vi "alignTop.vi"(8 "error in (no error)":errorcluster, 11 "refs":refnum<vi>[](array[refnum])) -> (0 "error out":errorcluster, 3 "refs(dup)":refnum<vi>[](array[refnum]))   [LabVIEW 2023, in "TLC_Geometry.lvlib"]
doc: "Aligns all controls to the topmost position among the input controls.\nThe topmost coordinate is computed and applied to all controls."
uses:
  TLC_Geometry.lvlib
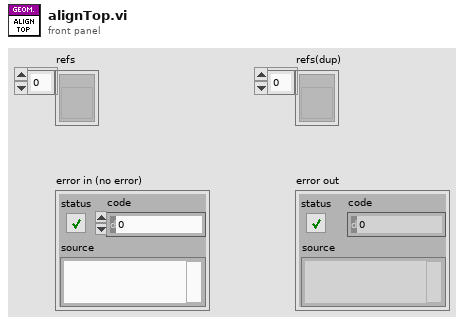
[diagram p1: front panel]
types:
  T1 = cluster{"left":i32, "top":i32, "right":i32, "bottom":i32}
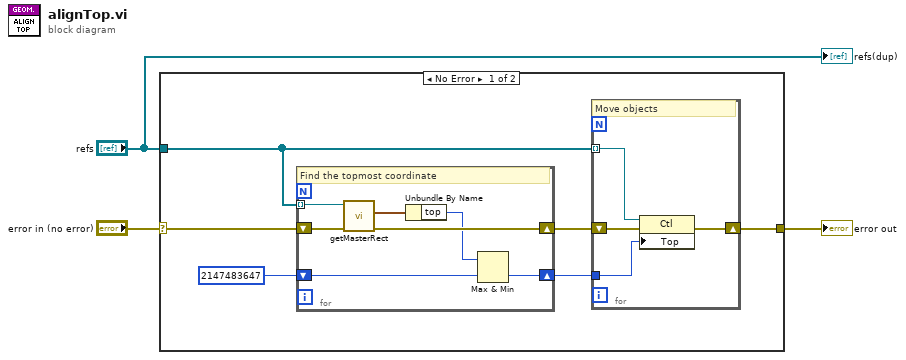
[diagram p0: block diagram]
diagram:
  n1 = case shown="No Error" "error in (no error)" {
    selector: "error in (no error)" -> [w9 w21]
    tunnel: [w6 w21] -> w2
    tunnel: "refs" -> [w7 _]
    frame No Error {
      n2 = for {
        tunnel: w7 -> [w20] mode=indexing
        shift-right: [w18] -> w5
        shift-left: w9 -> [w19]
        shift-right: [w15] -> w4
        shift-left: 2147483647 -> [w14]
        # "Find the topmost coordinate"
        n3 = call "getMasterRect.vi"("error in (no error)"=w19, "ref"=w20) -> ("error out"=w18:errorcluster, "rect"=w17:T1)  [unwired: 7 in, 1 out]
        n4 = Unbundle By Name(w17) -> ("top"=w16:i32)
        n5 = Max & Min(x=w16, y=w14) -> (min(x,y)=w15:i32)  [unwired: 1 out]
      }
      n6 = for {
        tunnel: w7 -> [w13] mode=indexing
        shift-right: [w11] -> w6
        shift-left: w5 -> [w12]
        tunnel: w4 -> [w10]
        # "Move objects"
        n7 = property class="Ctl"(reference=w13, error in=w12, "Top"=w10) -> (error out=w11:errorcluster)  [unwired: 1 out]
      }
    }
    frame Error {
    }
  }
  "error out" <- w2
  "refs(dup)" <- "refs"
